vi "WS1050_16 DUT VSA Save Data Ver1.0.vi"(0 "TMN DC\\CAP Data Log File Path":path=path "C:/temp", 1 "Lot#":string="WS1033", 2 "VSA_Delta C1(pF)":string[](array[string]), 4 "Wafer#":string="T4", 5 "File Name":string="Test Data", 6 "VSA_Delta C2(pF)":string[](array[string]), 7 "error in":errorcluster, 8 "Comment":string="Test Data", 9 "CP Current(uA)":string[](array[string]), 10 "VSA_IDD(A)":string="Test Data", 11 "HD Time(Min)":string="Test Data", 12 "Driver":string="Test Data", 13 "VSA_C1":string[](array[string]), 14 "CP HD (V)":string="Test Data", 15 "VSA_C2":string[](array[string]), 16 "SN":string[](array[string]), 17 "VSA_C3":string[](array[string]), 18 "Test Program":string="Test Data", 20 "Voltage(V)":string="Test Data", 21 "Stress Voltage(V)":string="Test Data", 26 "VSA_Delta C3(pF)":string[](array[string])) -> (27 "error out":errorcluster)   [LabVIEW 2012]
panel:
  # "*********** Do Not Remove ***********\nCompany:  WiSpry Inc\n20 Fairbanks Ste 198 Irvine CA 92618\n\nAuthor:  Andy V Tran\nCreated:  09/30/2014\nLabVIEW 2012 Suite\nTP:  Multi-Socket VSA CV Save Data\n*****************************************"
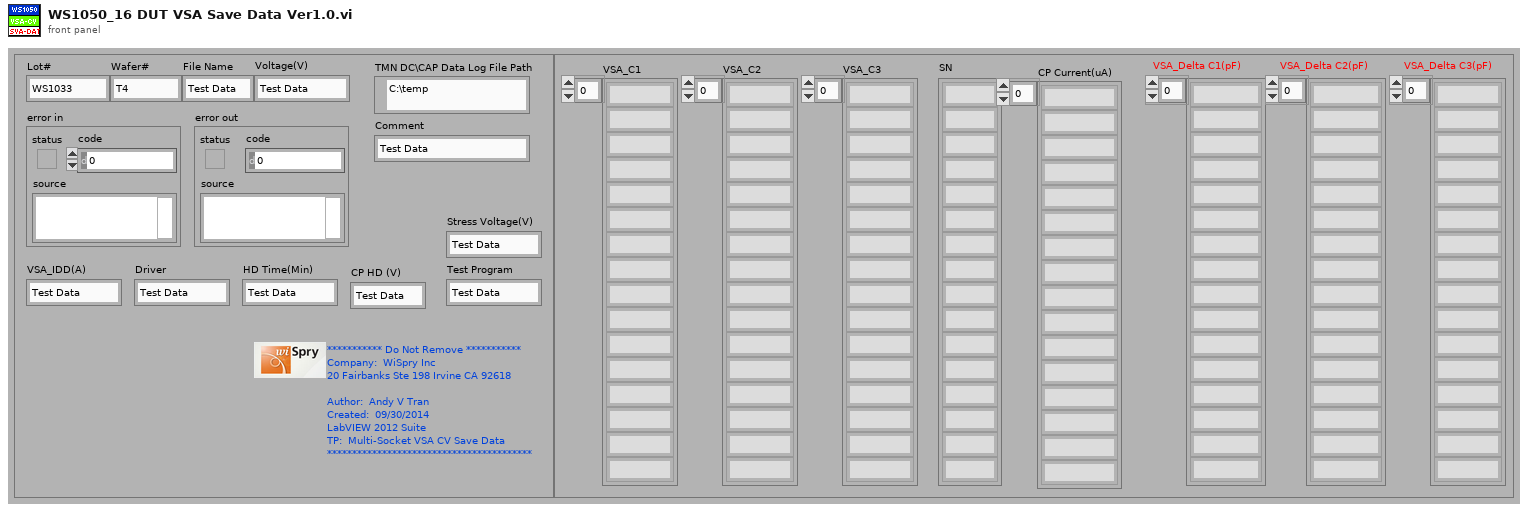
[diagram p1: front panel]
types:
  T1 = enum16{"open", "replace", "create", "open or create", "replace or create", "replace or create with confirmation"}
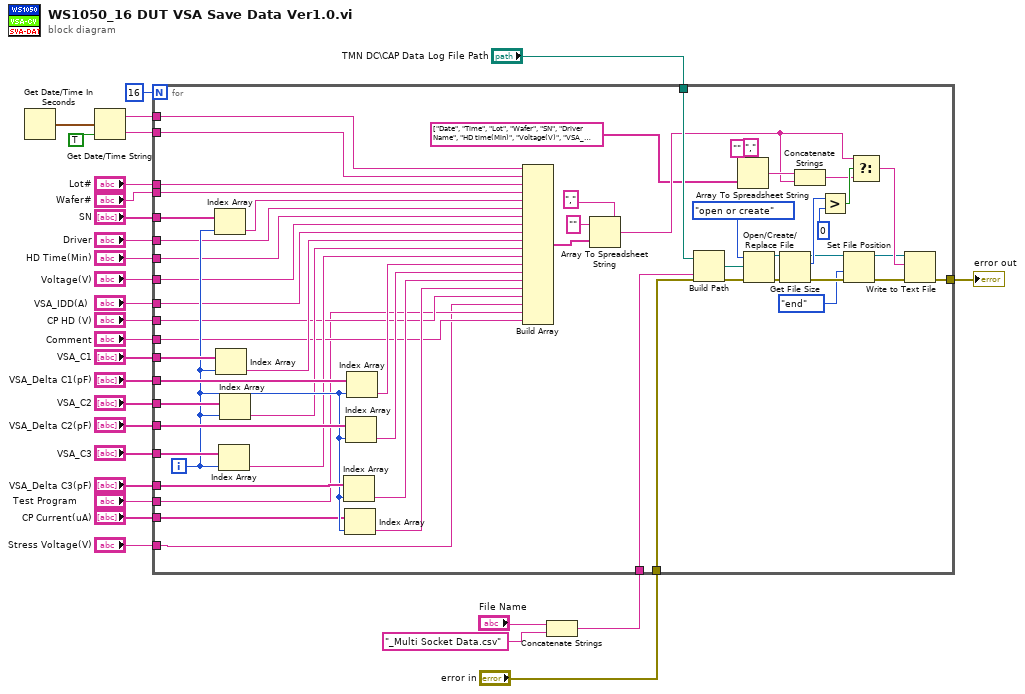
[diagram p0: block diagram]
diagram:
  n1 = Get Date/Time In Seconds() -> (seconds since 1Jan1904=w23:timestamp)
  n2 = Get Date/Time String(seconds (now)=w23, want seconds? (F)=TRUE) -> (date string=w21:string, time string=w20:string)  [unwired: 1 in]
  n3 = Concatenate Strings("File Name", "_Multi Socket Data.csv" ("string")) -> (w25:string)
  n4 = for {
    N: 16 -> [_]
    tunnel: "TMN DC\\CAP Data Log File Path" -> [w84]
    tunnel: "error in" -> [w83]
    tunnel: w25 -> [w82]
    tunnel: [w81] -> w24
    tunnel: w21 -> [w58]
    tunnel: w20 -> [w57]
    tunnel: "Lot#" -> [w56]
    tunnel: "Wafer#" -> [w55]
    tunnel: "SN" -> [w54]
    tunnel: "Voltage(V)" -> [w36]
    tunnel: "VSA_IDD(A)" -> [w37]
    tunnel: "Comment" -> [w32]
    tunnel: "VSA_C1" -> [w52]
    tunnel: "VSA_C2" -> [w51]
    tunnel: "VSA_C3" -> [w50]
    tunnel: "VSA_Delta C1(pF)" -> [w49]
    tunnel: "VSA_Delta C2(pF)" -> [w48]
    tunnel: "VSA_Delta C3(pF)" -> [w47]
    tunnel: "CP Current(uA)" -> [w45]
    tunnel: "HD Time(Min)" -> [w34]
    tunnel: "Driver" -> [w35]
    tunnel: "CP HD (V)" -> [w33]
    tunnel: "Test Program" -> [w31]
    tunnel: "Stress Voltage(V)" -> [w30]
    i -> [w46]
    n5 = Index Array(array=w54, index=w46) -> (element=w53:string)
    n6 = Index Array(array=w52, index=w46) -> (element=w38:string)
    n7 = Index Array(array=w50, index=w46) -> (element=w40:string)
    n8 = Index Array(array=w51, index=w46) -> (element=w39:string)
    n9 = Index Array(array=w47, index=w46) -> (element=w43:string)
    n10 = Index Array(array=w45, index=w46) -> (element=w44:string)
    n11 = Index Array(array=w48, index=w46) -> (element=w42:string)
    n12 = Index Array(array=w49, index=w46) -> (element=w41:string)
    n13 = Build Array(w58, w57, w56, w55, w53, w35, w34, w36, w37, w38, w39, w40, w41, w42, w43, w44, w33, w30, w31, w32) -> (w59:string[])
    n14 = Array To Spreadsheet String(delimiter (Tab)=",", array=w59, 3:"" ("format string")) -> (spreadsheet string=w61:string)
    n15 = Build Path(base path=w84, name or relative path=w82) -> (appended path=w75:path)
    n16 = Array To Spreadsheet String(delimiter (Tab)=",", array=string[] ["Date", "Time", "Lot", "Wafer", "SN", "Driver Name", "HD time(Min)", "Voltage(V)", "VSA_IDD(A)", "C1_(pF)", "C2_(pF)", "C3_(pF)", "Delta C1(pF)", "Delta C2(pF)", "Delta C3(pF)", "CP_IDD(uA)", "CP HD(V)", "Stress DCV(V)", "Test Program", "Comment"], 3:"" ("format string")) -> (spreadsheet string=w63:string)
    n17 = Open/Create/Replace File(file path (use dialog)=w75, error in=w83, operation (0:open)=T1."open or create") -> (refnum out=w73:refnum<file>, error out=w76:errorcluster)  [unwired: 4 out]
    n18 = Get File Size(file=w73, error in=w76) -> (refnum out=w68:refnum<file>, size (in bytes)=w72:i64, 0:w70:errorcluster)
    n19 = Concatenate Strings(w63, w61) -> (w62:string)
    n20 = Greater?(x=w72, y=i64 0) -> (0:w77:bool)
    n21 = Set File Position(refnum=w68, from (0:start)=enum16{"start", "end", "current"}."end", error in=w70) -> (refnum out=w67:refnum<file>, error out=w69:errorcluster)  [unwired: 1 out]
    n22 = Select(t=w61, s=w77, f=w62) -> (s? t:f=w74:string)
    n23 = Write to Text File(file (use dialog)=w67, text=w74, error in=w69) -> (error out=w81:errorcluster)  [unwired: 3 out]
  }
  "error out" <- w24
